vi "替换1（10替换）.vi"(1 "改变的数组":i32[][](array[numeric]), 2 "检索的数组":i32[][](array[numeric])) -> (0 "显示 2":i32[][](array[numeric]))   [LabVIEW 2014]
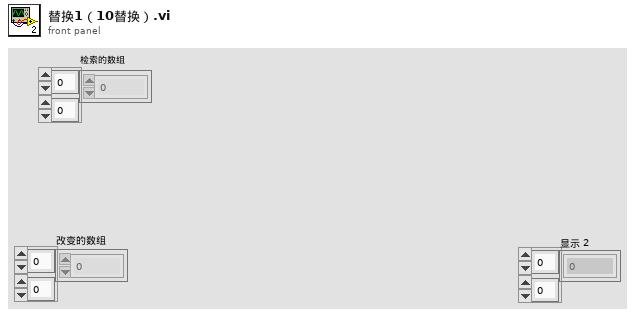
[diagram p1: front panel]
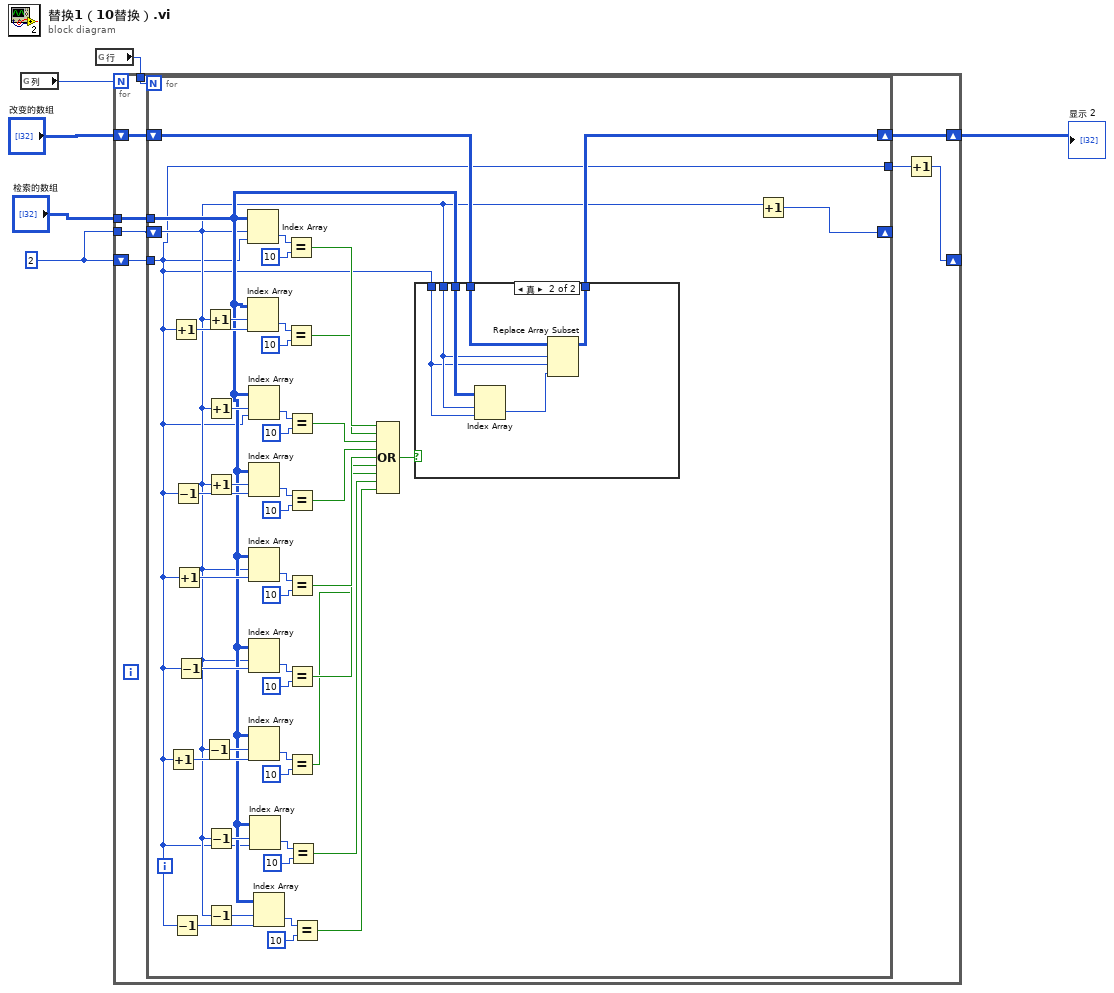
[diagram p0: block diagram]
diagram:
  w6 = 2
  n1 = global read "全局 1.vi" "列"() -> (w3:i32)
  n2 = global read "全局 1.vi" "行"() -> (w2:i32)
  n3 = for {
    N: w3 -> [_]
    tunnel: "检索的数组" -> [w14]
    tunnel: w6 -> [w11]
    shift-right: [w13] -> w4
    shift-left: "改变的数组" -> [w12]
    shift-right: [w8] -> _
    shift-left: w6 -> [w9]
    tunnel: w2 -> [w7]
    n4 = for {
      N: w7 -> [_]
      tunnel: w14 -> [w20]
      tunnel: w9 -> [w15]
      shift-right: [w19] -> w13
      shift-left: w12 -> [w18]
      shift-right: [w17] -> _
      shift-left: w11 -> [w16]
      tunnel: [w15] -> w10
      n5 = Increment(x=w15) -> (x+1=w32:i32)
      n6 = Increment(x=w15) -> (x+1=w39:i32)
      n7 = Decrement(x=w15) -> (x-1=w31:i32)
      n8 = Decrement(x=w15) -> (x-1=w38:i32)
      n9 = Increment(x=w15) -> (x+1=w37:i32)
      n10 = Decrement(x=w15) -> (x-1=w36:i32)
      n11 = Decrement(x=w16) -> (x-1=w35:i32)
      n12 = Increment(x=w16) -> (x+1=w42:i32)
      n13 = Increment(x=w16) -> (x+1=w40:i32)
      n14 = Increment(x=w16) -> (x+1=w41:i32)
      n15 = Decrement(x=w16) -> (x-1=w34:i32)
      n16 = Decrement(x=w16) -> (x-1=w33:i32)
      n17 = Index Array(array=w20, index (row)=w16, index (col)=w15) -> (element=w60:i32)
      n18 = Index Array(array=w20, index (row)=w42, index (col)=w39) -> (element=w58:i32)
      n19 = Index Array(array=w20, index (row)=w40, index (col)=w15) -> (element=w56:i32)
      n20 = Index Array(array=w20, index (row)=w41, index (col)=w38) -> (element=w54:i32)
      n21 = Index Array(array=w20, index (row)=w16, index (col)=w37) -> (element=w52:i32)
      n22 = Index Array(array=w20, index (row)=w16, index (col)=w36) -> (element=w50:i32)
      n23 = Index Array(array=w20, index (row)=w35, index (col)=w32) -> (element=w48:i32)
      n24 = Index Array(array=w20, index (row)=w34, index (col)=w15) -> (element=w46:i32)
      n25 = Index Array(array=w20, index (row)=w33, index (col)=w31) -> (element=w44:i32)
      n26 = Equal?(x=w60, y=10) -> (x = y?=w30:bool)
      n27 = Equal?(x=w58, y=10) -> (x = y?=w29:bool)
      n28 = Equal?(x=w56, y=10) -> (x = y?=w28:bool)
      n29 = Equal?(x=w54, y=10) -> (x = y?=w27:bool)
      n30 = Equal?(x=w52, y=10) -> (x = y?=w26:bool)
      n31 = Equal?(x=w50, y=10) -> (x = y?=w25:bool)
      n32 = Equal?(x=w48, y=10) -> (x = y?=w24:bool)
      n33 = Equal?(x=w46, y=10) -> (x = y?=w23:bool)
      n34 = Equal?(x=w44, y=10) -> (x = y?=w22:bool)
      n35 = Compound Arithmetic op=OR(w30, w29, w28, w27, w26, w25, w24, w23, w22) -> (w21:bool)
      n36 = case shown="真" w21 {
        tunnel: w18 -> [w61 w67]
        tunnel: w20 -> [_ w66]
        tunnel: w15 -> [_ w63]
        tunnel: w16 -> [_ w64]
        tunnel: [w61 w62] -> w19
        frame False {
        }
        frame True {
          n37 = Index Array(array=w66, index (row)=w64, index (col)=w63) -> (element=w65:i32)
          n38 = Replace Array Subset(array=w67, new element=w65, index (row)=w64, index (col)=w63) -> (w62:i32[][])
        }
      }
      n39 = Increment(x=w16) -> (x+1=w17:i32)
    }
    n40 = Increment(x=w10) -> (x+1=w8:i32)
  }
  "显示 2" <- w4
